vi "testbed.vi"() -> ()   [LabVIEW 2020]
uses:
  _libraries/Path Utilities/Path Utilities.lvlib
  toolbox/Timing/Timing.lvlib
  toolbox/User Interface/User Interface.lvlib
  toolbox/Debugging/Debugging.lvlib
  _libraries/Config Data/Config Data.lvclass
  _libraries/Display Properties Manager/Display Properties Manager.lvlib
panel:
  out "progress":string
  out "error out":errorcluster
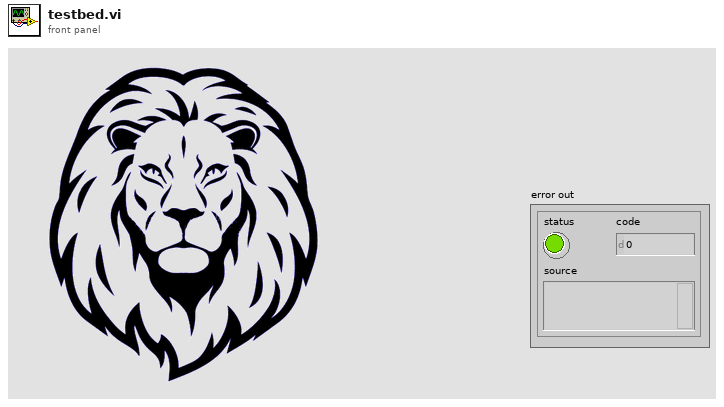
[diagram p1: front panel]
types:
  T1 = typedef "Config Data.lvlib/Config Data.lvclass/Process Launch Data.ctl" = cluster{"Label":string, "File Path":path, "Launch Mode":T2}
  T2 = typedef "Config Data.lvlib/Config Data.lvclass/Process Type.ctl" = enum16{"Async - Non-Reentrant", "Async - Reentrant", "Run Method - Non-Reentrant", "Run Method - Reentrant"}
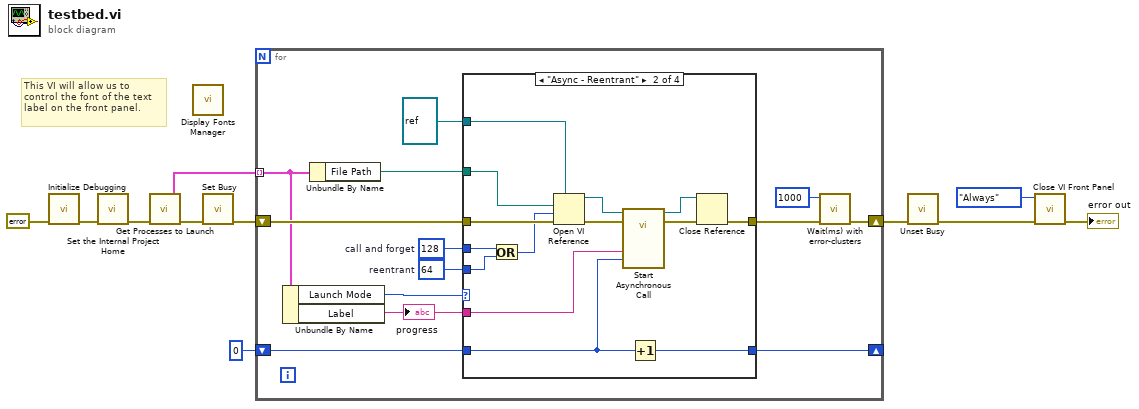
[diagram p0: block diagram]
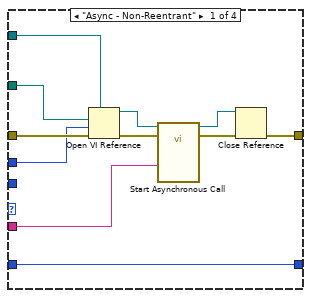
[diagram p2: hidden frame]
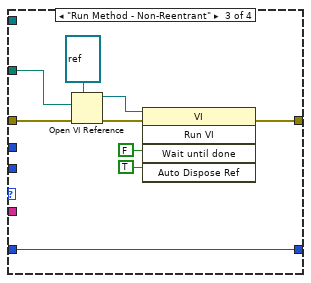
[diagram p3: hidden frame]
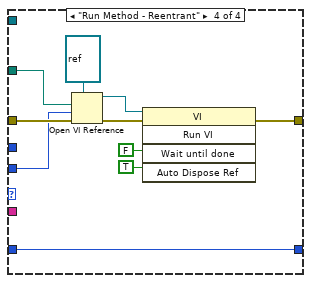
[diagram p4: hidden frame]
diagram:
  # "This VI will allow us to control the font of the text label on the front panel."
  n1 = call "Initialize Debugging.vi"("Error In"=errorcluster {"status"=FALSE, "code"=0, "source"=""} ("error in (no error)")) -> ("Error Out"=w2:errorcluster)  [unwired: 6 in]
  n2 = call "Set the Internal Project Home.vi"("Error In"=w2) -> ("Error Out"=w10:errorcluster)  [unwired: 6 in]
  n3 = call "Get Processes to Launch.vi"("Error In"=w10) -> ("Error Out"=w9:errorcluster, "Processes to Launch"=w11:T1[])  [unwired: 5 in]
  n4 = call "Display Fonts Manager.vi"() -> ()  [unwired: 7 in, 1 out]
  n5 = call <vilib>:"Set Busy.vi"("error in (no error)"=w9) -> ("error out"=w8:errorcluster)  [unwired: 9 in, 1 out]
  n6 = for {
    shift-right: [w18] -> w7
    shift-left: w8 -> [w24]
    tunnel: w11 -> [w23] mode=indexing
    shift-right: [w12] -> _
    shift-left: 0 -> [w13]
    w14 = 64  # reentrant
    w22 = 128  # call and forget
    n7 = Unbundle By Name(w23) -> ("Launch Mode"=w21:T2, "Label"=w16:string)
    "progress" <- w16
    n8 = Unbundle By Name(w23) -> ("File Path"=w20:path)
    n9 = case shown="\"Async - Reentrant\"" w21 {
      tunnel: w24 -> [w35 w49 w58 w68]
      tunnel: w20 -> [w34 w48 w57 w67]
      tunnel: w22 -> [w31 w42 _ _]
      tunnel: [w28 w43 w51 w61] -> w19
      tunnel: w16 -> [w27 w40 _ _]
      tunnel: refnum<vi> refnum ("type specifier VI Refnum (for type only)") -> [w26 w39 _ _]
      tunnel: w14 -> [_ w38 _ w60]
      tunnel: w13 -> [w25 w37 w50 w59]
      tunnel: [w25 w36 w50 w59] -> w12
      frame "Async - Non-Reentrant" {
        n10 = Open VI Reference(type specifier VI Refnum (for type only)=w26, vi path=w34, options=w31, error in (no error)=w35) -> (vi reference=w33:refnum<vi>, error out=w32:errorcluster)  [unwired: 2 in]
        n11 = call-by-ref "Start Asynchronous Call"(reference=w33, error in=w32, "My Name"=w27) -> (reference out=w29:refnum<vi>, error out=w30:errorcluster)  [unwired: 11 in]
        n12 = Close Reference(reference=w29, error in (no error)=w30) -> (error out=w28:errorcluster)
      }
      frame "Async - Reentrant" {
        n13 = Or(x=w42, y=w38) -> (x .or. y?=w41:i32)
        n14 = Open VI Reference(type specifier VI Refnum (for type only)=w39, vi path=w48, options=w41, error in (no error)=w49) -> (vi reference=w47:refnum<vi>, error out=w46:errorcluster)  [unwired: 2 in]
        n15 = call-by-ref "Start Asynchronous Call"(reference=w47, error in=w46, "Launch Order"=w37, "My Name"=w40) -> (reference out=w44:refnum<vi>, error out=w45:errorcluster)  [unwired: 10 in]
        n16 = Increment(x=w37) -> (x+1=w36:i32)
        n17 = Close Reference(reference=w44, error in (no error)=w45) -> (error out=w43:errorcluster)
      }
      frame "Run Method - Non-Reentrant" {
        n18 = Open VI Reference(type specifier VI Refnum (for type only)=refnum<vi> refnum, vi path=w57, error in (no error)=w58) -> (vi reference=w55:refnum<vi>, error out=w54:errorcluster)  [unwired: 3 in]
        n19 = invoke class="VI" method="Run VI"(reference=w55, error in=w54, "Wait until done"=FALSE ("Wait Until Done"), "Auto Dispose Ref"=TRUE ("Wait Until Done")) -> (error out=w51:errorcluster)  [unwired: 1 in, 4 out]
      }
      frame "Run Method - Reentrant" {
        n20 = Open VI Reference(type specifier VI Refnum (for type only)=refnum<vi> refnum, vi path=w67, options=w60, error in (no error)=w68) -> (vi reference=w65:refnum<vi>, error out=w64:errorcluster)  [unwired: 2 in]
        n21 = invoke class="VI" method="Run VI"(reference=w65, error in=w64, "Wait until done"=FALSE ("Wait Until Done"), "Auto Dispose Ref"=TRUE ("Wait Until Done")) -> (error out=w61:errorcluster)  [unwired: 1 in, 4 out]
      }
    }
    n22 = call "Wait(ms) with error-clusters.vi"("Error In"=w19, "wait (msec)"=u32 1000 ("milliseconds to wait")) -> ("Error Out"=w18:errorcluster)  [unwired: 5 in]
  }
  n23 = call <vilib>:"Unset Busy.vi"("error in (no error)"=w7) -> ("error out"=w4:errorcluster)  [unwired: 10 in]
  n24 = call "Close VI Front Panel.vi"("Error In"=w4, "When"=enum16{"Always", "Not Development"}."Always") -> ("Error Out"=→"error out":errorcluster)  [unwired: 5 in]
